vi "thesis plots.vi"() -> ()   [LabVIEW 2010]
panel:
  out "DOS PLot":cluster{dbl[], dbl[]}[](graph)
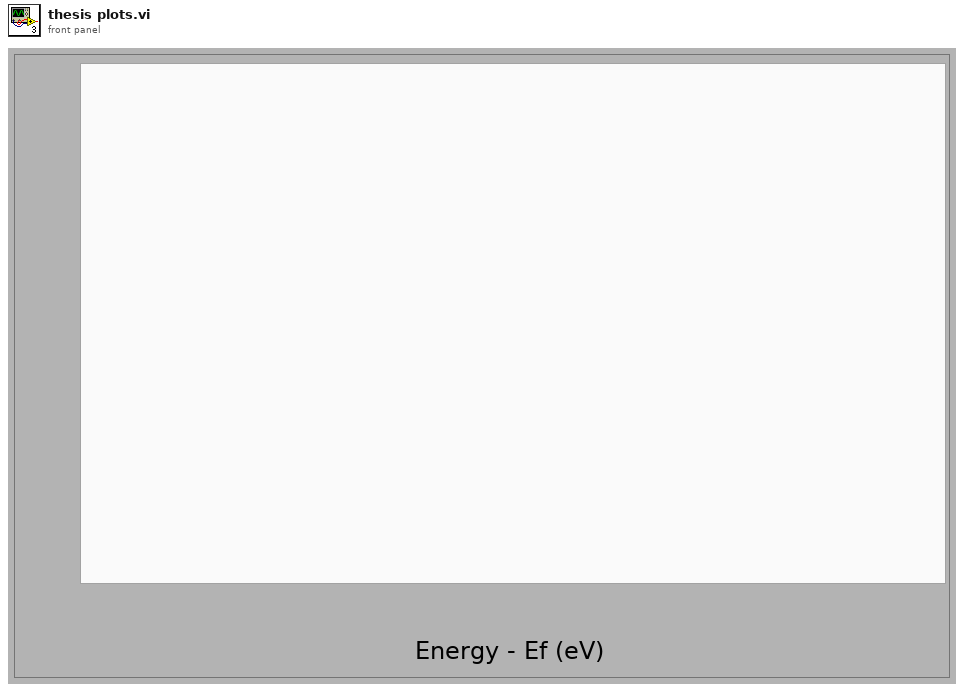
[diagram p1: front panel]
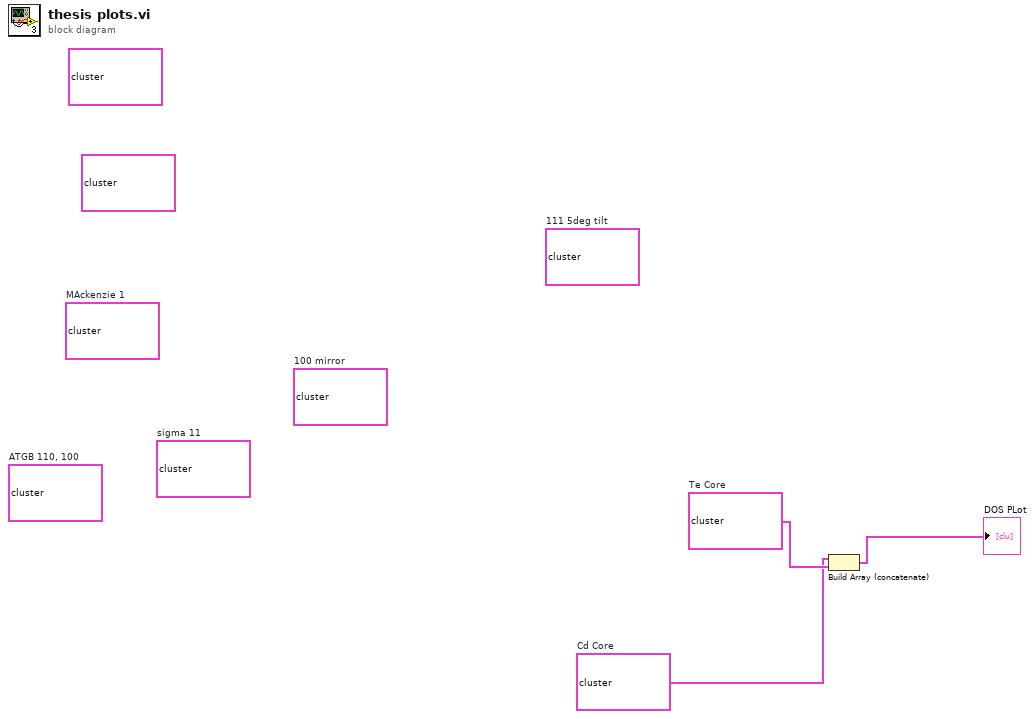
[diagram p0: block diagram]
diagram:
  w2 = cluster{dbl[], dbl[]}[] [{array[2000 elements], array[2000 elements]}, {array[2000 elements], array[2000 elements]}]  # Cd Core
  w3 = cluster{dbl[], dbl[]}[] [{array[2000 elements], array[2000 elements]}, {array[2000 elements], array[2000 elements]}]  # Te Core
  (unwired) cluster{dbl[], dbl[]}[] [{array[2000 elements], array[2000 elements]}, {array[2000 elements], array[2000 elements]}]  # ATGB 110, 100
  (unwired) cluster{dbl[], dbl[]}[] [{array[2000 elements], array[2000 elements]}, {array[2000 elements], array[2000 elements]}]  # MAckenzie 1
  (unwired) cluster{dbl[], dbl[]}[] [{array[2000 elements], array[2000 elements]}, {array[2000 elements], array[2000 elements]}]  # sigma 11
  (unwired) cluster{dbl[], dbl[]}[] [{array[2000 elements], array[2000 elements]}, {array[2000 elements], array[2000 elements]}]  # 111 5deg tilt
  (unwired) cluster{dbl[], dbl[]}[] [{array[2000 elements], array[2000 elements]}, {array[2000 elements], array[2000 elements]}]  # 100 mirror
  (unwired) cluster{dbl[], dbl[]}[] [{array[2000 elements], array[2000 elements]}, {array[2000 elements], array[2000 elements]}] ("DOS PLot 2")
  (unwired) cluster{dbl[], dbl[]}[] [{array[2000 elements], array[2000 elements]}, {array[2000 elements], array[2000 elements]}] ("DOS PLot 2")
  n1 = Build Array (concatenate)(w2, w3) -> (→"DOS PLot":cluster{dbl[], dbl[]}[])
